vi "1xSTRING_Int.vi"() -> ()   [LabVIEW 2015]
uses:
  <vilib>/Platform/TimedLoop/XDataNode/XDataNode.xnode
  <vilib>/Platform/TimedLoop/XDataNode/nitl_modes.ctl
  <vilib>/Platform/TimedLoop/XDataNode/XDNodeRunTimeDep.lvlib
  <vilib>/Platform/TimedLoop/XDataNode/wakeup.ctl
  <vilib>/Platform/TimedLoop/XDataNode/timing_clust.ctl
  <vilib>/rvi/DataTransferAndStorage/Container/XNode/niFpgaContainer.xnode
  <vilib>/eio/EIONode/EIONode.xnode
  <vilib>/rvi/eio/common/nirviEmuTemplateMethod_errors.vi
  <vilib>/rvi/Memory/Memory_Emulation/nirvimemoryEmulation.vi
  <vilib>/rvi/Memory/Memory_Emulation/nirvimemoryFastEmulation.vi
  <vilib>/rvi/interface/RandomDataEmulation/nirviRandomDataFpgaReadWriteTemplate.vi
  <vilib>/rvi/FIFO/Fifo_Resource/nirvififoEmulationWrite.vi
  <vilib>/rvi/FIFO/Fifo_Resource/nirvififoEmulationRead.vi
panel:
  in  "1/2":bool
  in  "Scale":i8
  in  "Levels":u8
  in  "Delay?":bool
  in  "1/Attack":fxp<+,16,0>
  in  "1/Decay":fxp<+,16,0>
  in  "Sustain":fxp<+,16,0>
  in  "S/R":fxp<+,16,0>
  in  "Amount":fxp<+,8,0>
  in  "Gate":bool
  in  "LFO":fxp<+/-,8,8>
  out "VCA Out":i16
  in  "Init?":bool
  out "From Host?":bool
  out "To Host?":bool
  in  "Start":bool
  out "Recording":bool
  in  "Clear?":bool
  out "Flag":bool
  in  "Transfer":bool
  in  "M":fxp<+,32,32>
  in  "Trigger":bool
  # "VCO"
  # "VCA"
  # "Rep"
  # "Interf"
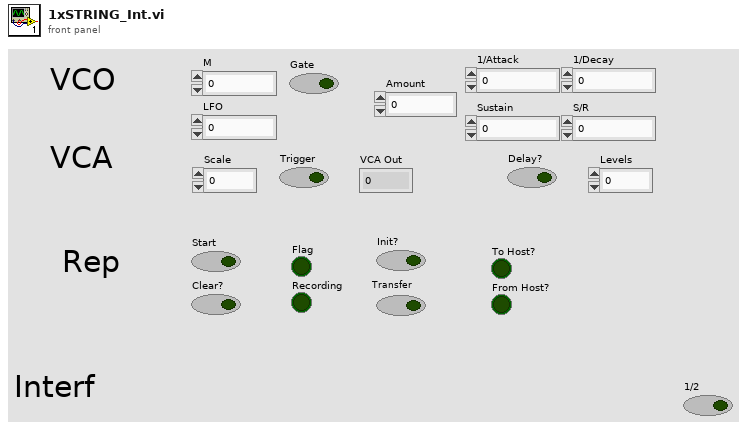
[diagram p1: front panel]
types:
  T1 = typedef "XDNodeRunTimeDep.lvlib/timing_clust.ctl" = cluster{"Expected End [f-1]":u64, "Actual End [f-1]":u64, "Finished Late? [f-1]":bool, "Expected End [i-1]":u64, "Actual End [i-1]":u64, "Finished Late? [i-1]":bool, "Expected Start [i]":u64, "Actual Start [i]":u64, "Expected Start [f]":u64, "Actual Start [f]":u64, "Source Name":string, "Structure Name":string, "Period":i64, "Deadline":i64, "Offset":i64, "Start":i64, "Priority":i32, "Timeout":i32, "Mode":T2, "Wakeup Reason":T3, "Error":errorcluster, "Source Type":string, "Secondary Source Type":string, "Global End Time":u64, "Global Start Time":u64, "Frame Duration":u64, "Iteration Duration":u64, "Assigned CPU":i32, "I/O Scan Engine Mode":u32}
  T2 = typedef "XDNodeRunTimeDep.lvlib/nitl_modes.ctl" = enum32{"No Change", "Process missed periods, maintain original phase", "Discard missed periods, maintain original phase", "Process missed periods, ignore original phase", "Discard missed periods, ignore original phase"}
  T3 = typedef "XDNodeRunTimeDep.lvlib/wakeup.ctl" = enum32{"Normal", "Aborted", "Asynchronous wakeup", "Timing source error", "Timed loop error", "Timeout"}
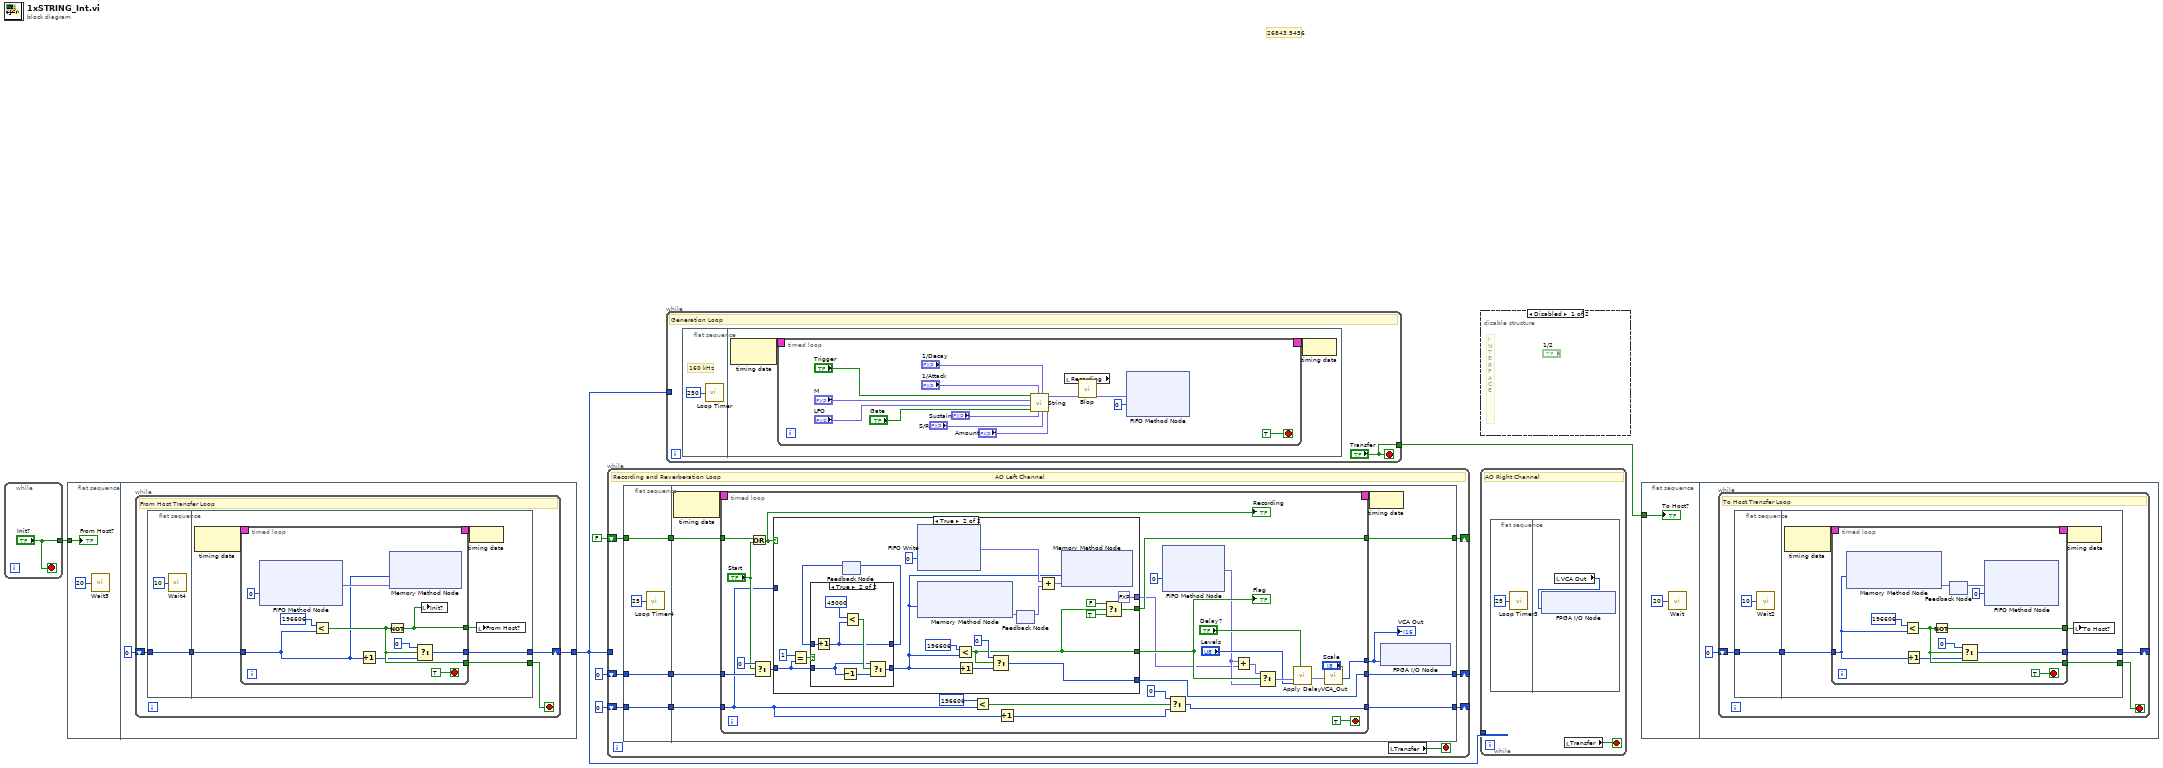
[diagram p0: block diagram]
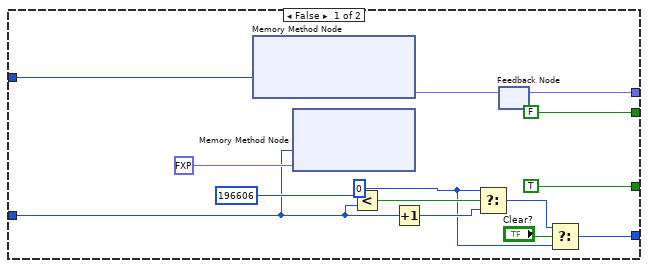
[diagram p3: hidden frame]
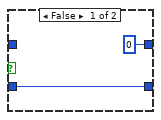
[diagram p4: hidden frame]
diagram:
  # "26843,5456"
  n1 = while {
    tunnel: ["Init?"] -> w4
    stop <- "Init?" stop-if-true
  }
  n2 = flat-sequence {
    tunnel: w4 -> [w9]
    tunnel: [w10] -> w3
    frame #0 {
      n3 = call "Wait3"("Count(mSec)"=u8 20) -> ()  [unwired: 1 out]
      "From Host?" <- w9
    }
    frame #1 {
      n4 = while {
        shift-right: [w13] -> w10
        shift-left: u32 0 -> [w14]
        stop <- w12 stop-if-true
        # "From Host Transfer Loop"
        n5 = flat-sequence {
          tunnel: [w17] -> w15
          tunnel: w14 -> [w17]
          tunnel: w15 -> [w21]
          tunnel: [w20] -> w13
          tunnel: [w19] -> w12
          frame #0 {
            n6 = call "Wait4"("Count(uSec)"=u8 10) -> ()  [unwired: 1 out]
          }
          frame #1 {
            n7 = node-c288() -> (w23:T1)  [unwired: 1 in]
            n8 = timed-loop {
              timing: w23 -> [_]
              timing-out: [_] -> w22
              tunnel: w21 -> [w26]
              tunnel: [w29] -> w19
              tunnel: [w28] -> w20
              tunnel: [w24] -> w18
              stop <- TRUE stop-if-true
              n9 = xnode ("FIFO Method Node")("Timeout"=0) -> ("Element"=w33:fxp<+/-,8,8>)  [unwired: 1 in, 2 out]
              n10 = Less?(x=u32 196606, y=w26) -> (x < y?=w29:bool)
              n11 = Increment(x=w26) -> (x+1=w25:u32)
              n12 = Not(x=w29) -> (.not. x?=w24:bool)
              n13 = xnode ("Memory Method Node")("Address"=w26, "Data"=w33) -> ()  [unwired: 1 in, 1 out]
              n14 = Select(t=u32 0, s=w29, f=w25) -> (s? t:f=w28:u32)
              n15 = local write "Init?"(w24) -> ()
            }
            n16 = node-c288(w22) -> ()
            n17 = local write "From Host?"(w18) -> ()
          }
        }
      }
    }
  }
  n18 = while {
    shift-right: [w38] -> _
    shift-left: u32 0 ("Address") -> [w46]
    shift-right: [w43] -> _
    shift-left: FALSE ("t") -> [w44]
    tunnel: w3 -> [_]
    shift-right: [w39] -> _
    shift-left: u32 0 ("Address") -> [w40]
    stop <- w42 stop-if-true
    # "Recording and Reverberation Loop                                                                                                                                         AO Left Channel"
    n19 = flat-sequence {
      tunnel: [w50] -> w47
      tunnel: w46 -> [w50]
      tunnel: w44 -> [w49]
      tunnel: [w49] -> w45
      tunnel: [w48] -> w41
      tunnel: w40 -> [w48]
      tunnel: w47 -> [w60]
      tunnel: w45 -> [w59]
      tunnel: [w58] -> w43
      tunnel: w41 -> [w55]
      tunnel: [w54] -> w39
      tunnel: [w52] -> w38
      frame #0 {
        n20 = call "Loop Timer4"("Count(uSec)"=u8 25) -> ()  [unwired: 1 out]
      }
      frame #1 {
        n21 = node-c288() -> (w57:T1)  [unwired: 1 in]
        n22 = timed-loop {
          timing: w57 -> [_]
          timing-out: [_] -> w56
          tunnel: w60 -> [w71]
          tunnel: w59 -> [w69]
          tunnel: [w67] -> w58
          tunnel: w55 -> [w62]
          tunnel: [w75] -> w54
          tunnel: [w74] -> w53
          tunnel: [w65] -> w52
          stop <- TRUE stop-if-true
          n23 = Or(x=w69, y="Start") -> (x .or. y?=w68:bool)
          "Recording" <- w68
          n24 = Select(t=u32 0, s="Start", f=w71) -> (s? t:f=w72:u32)
          n25 = case shown="True" w68 {
            tunnel: [w100 w112] -> w65
            tunnel: w72 -> [w94 w106]
            tunnel: [FALSE ("t") w119] -> w67
            tunnel: [TRUE w109] -> w66
            tunnel: w62 -> [w92 _]
            tunnel: [w90 fxp<+/-,8,8> 0.0 ("Data")] -> w61
            frame False {
              w89 = u32 0 ("y")
              n26 = xnode ("Memory Method Node")("Address"=w92) -> ("Data"=w91:fxp<+/-,8,8>)  [unwired: 1 in, 1 out]
              n27 = xnode ("Memory Method Node")("Address"=w94, "Data"=fxp<+/-,8,8> 0.0) -> ()  [unwired: 1 in, 1 out]
              n28 = Less?(x=u32 196606 ("y"), y=w94) -> (x < y?=w99:bool)
              n29 = Increment(x=w94) -> (x+1=w95:u32)
              n30 = Select(t=w89, s=w99, f=w95) -> (s? t:f=w97:u32)
              n31 = feedback #1() -> (w90:fxp<+/-,8,8>)  [unwired: 1 in]
              n32 = feedback-in #1(w91) -> ()
              n33 = Select(t=w97, s="Clear?", f=w89) -> (s? t:f=w100:u32)
            }
            frame True {
              n34 = Equal?(x=u32 1, y=w106) -> (x = y?=w107:bool)
              n35 = feedback #2() -> (w103:u32)  [unwired: 1 in]
              n36 = case shown="True" w107 {
                tunnel: w106 -> [w122 w124]
                tunnel: [w122 w128] -> w105
                tunnel: [u32 0 w123] -> w104
                tunnel: w103 -> [_ w129]
                frame False {
                }
                frame True {
                  n37 = Increment(x=w129) -> (x+1=w123:u32)
                  n38 = Decrement(x=w124) -> (x-1=w125:u32)
                  n39 = Less?(x=u32 45000 ("End"), y=w123) -> (x < y?=w126:bool)
                  n40 = Select(t=w124, s=w126, f=w125) -> (s? t:f=w128:u32)
                }
              }
              n41 = feedback-in #2(w104) -> ()
              n42 = xnode ("FIFO Write")("Timeout"=0) -> ("Element"=w115:fxp<+/-,8,8>)  [unwired: 1 in, 2 out]
              n43 = xnode ("Memory Method Node")("Address"=w105) -> ("Data"=w113:fxp<+/-,8,8>)  [unwired: 1 in, 1 out]
              n44 = Less?(x=u32 196606 ("y"), y=w105) -> (x < y?=w109:bool)
              n45 = Increment(x=w105) -> (x+1=w116:u32)
              n46 = Select(t=u32 0, s=w109, f=w116) -> (s? t:f=w112:u32)
              n47 = feedback-in #3(w113) -> ()
              n48 = feedback #3() -> (w110:fxp<+/-,8,8>)  [unwired: 1 in]
              n49 = Add(x=w115, y=w110) -> (x+y=w114:fxp<+/-,8,8>)
              n50 = xnode ("Memory Method Node")("Address"=w105, "Data"=w114) -> ()  [unwired: 1 in, 1 out]
              n51 = Select(t=FALSE, s=w109, f=TRUE) -> (s? t:f=w119:bool)
            }
          }
          "Flag" <- w66
          n52 = Less?(x=u32 196606, y=w62) -> (x < y?=w78:bool)
          n53 = Increment(x=w62) -> (x+1=w80:u32)
          n54 = xnode ("FIFO Method Node")("Timeout"=0) -> ("Element"=w63:fxp<+/-,8,8>)  [unwired: 1 in, 2 out]
          n55 = Select(t=u32 0, s=w78, f=w80) -> (s? t:f=w75:u32)
          n56 = Add(x=w63, y=w61) -> (x+y=w64:fxp<+/-,8,8>)
          n57 = Select(t=w64, s=w66, f=w63) -> (s? t:f=w84:fxp<+/-,8,8>)
          n58 = call "Apply Delay.vi"("Delay?"="Delay?", "Levels"="Levels", "Element in"=w84) -> ("Element out"=w85:fxp<+/-,8,8>)  [unwired: 8 in]
          n59 = call "VCA_Out.vi"("Scale"="Scale", "Sample In"=w85) -> ("Sample Out"=w74:i16)  [unwired: 9 in]
        }
        "VCA Out" <- w53
        n60 = node-c288(w56) -> ()
        n61 = xnode "FPGA I/O Node"("AudioOut/Left"=w53) -> ()  [unwired: 1 in, 1 out]
      }
    }
    n62 = local read "Transfer"() -> (w42:bool)
  }
  n63 = while {
    tunnel: w3 -> [_]
    tunnel: ["Transfer"] -> w1
    stop <- "Transfer" stop-if-true
    # "Generation Loop"
    n64 = flat-sequence {
      frame #0 {
        # "160 kHz"
        n65 = call "Loop Timer"("Count(Ticks)"=u8 250) -> ()  [unwired: 1 out]
      }
      frame #1 {
        n66 = node-c288() -> (w137:T1)  [unwired: 1 in]
        n67 = timed-loop {
          timing: w137 -> [_]
          timing-out: [_] -> w136
          stop <- TRUE stop-if-true
          n68 = call "String.vi"("Amount"="Amount", "S/R"="S/R", "1/Decay"="1/Decay", "Sustain"="Sustain", "1/Attack"="1/Attack", "Gate"="Gate", "LFO"="LFO", "M"="M", "Trigger"="Trigger") -> ("String Out"=w147:fxp<+/-,8,8>)  [unwired: 2 in]
          n69 = local read "Recording"() -> (w148:bool)
          n70 = call "Blop.vi"("Rec"=w148, "Sample In"=w147) -> ("Sample Out"=w149:fxp<+/-,8,8>)  [unwired: 9 in]
          n71 = xnode ("FIFO Method Node")("Element"=w149, "Timeout"=0) -> ()  [unwired: 1 in, 2 out]
        }
        n72 = node-c288(w136) -> ()
      }
    }
  }
  n73 = disable-structure shown="Disabled" {
    frame Disabled {
      # "I\nN\nT\nE\nR\nF\nA\nC\nE"
    }
    frame Enabled {
    }
  }
  n74 = while {
    tunnel: w3 -> [_]
    stop <- w156 stop-if-true
    # "AO Right Channel"
    n75 = flat-sequence {
      frame #0 {
        n76 = call "Loop Timer3"("Count(uSec)"=u8 25) -> ()  [unwired: 1 out]
      }
      frame #1 {
        n77 = local read "VCA Out"() -> (w158:i16)
        n78 = xnode "FPGA I/O Node"("AudioOut/Right"=w158) -> ()  [unwired: 1 in, 1 out]
      }
    }
    n79 = local read "Transfer"() -> (w156:bool)
  }
  n80 = flat-sequence {
    tunnel: w1 -> [w160]
    frame #0 {
      n81 = call "Wait"("Count(mSec)"=u8 20) -> ()  [unwired: 1 out]
      "To Host?" <- w160
    }
    frame #1 {
      n82 = while {
        shift-right: [w163] -> _
        shift-left: u32 0 -> [w164]
        stop <- w162 stop-if-true
        # "To Host Transfer Loop"
        n83 = flat-sequence {
          tunnel: [w167] -> w165
          tunnel: w164 -> [w167]
          tunnel: w165 -> [w171]
          tunnel: [w170] -> w163
          tunnel: [w169] -> w162
          frame #0 {
            n84 = call "Wait2"("Count(uSec)"=u8 10) -> ()  [unwired: 1 out]
          }
          frame #1 {
            n85 = node-c288() -> (w173:T1)  [unwired: 1 in]
            n86 = timed-loop {
              timing: w173 -> [_]
              timing-out: [_] -> w172
              tunnel: w171 -> [w177]
              tunnel: [w182] -> w169
              tunnel: [w181] -> w170
              tunnel: [w174] -> w168
              stop <- TRUE stop-if-true
              n87 = xnode ("Memory Method Node")("Address"=w177) -> ("Data"=w176:fxp<+/-,8,8>)  [unwired: 1 in, 1 out]
              n88 = Less?(x=u32 196606, y=w177) -> (x < y?=w182:bool)
              n89 = Increment(x=w177) -> (x+1=w179:u32)
              n90 = Not(x=w182) -> (.not. x?=w174:bool)
              n91 = feedback-in #4(w176) -> ()
              n92 = feedback #4() -> (w175:fxp<+/-,8,8>)  [unwired: 1 in]
              n93 = Select(t=u32 0, s=w182, f=w179) -> (s? t:f=w181:u32)
              n94 = xnode ("FIFO Method Node")("Element"=w175, "Timeout"=0) -> ()  [unwired: 1 in, 2 out]
            }
            n95 = node-c288(w172) -> ()
            n96 = local write "To Host?"(w168) -> ()
          }
        }
      }
    }
  }
